vi "Fetch_Source.vi"(8 "error in (no error)":errorcluster, 9 "destTag":string, 10 "sourceTag":string, 11 "Installer in":refnum<class "Installer.lvclass">) -> (0 "error out":errorcluster, 2 "index":i32, 3 "IB_Source.lvclass":refnum<class "IB_Source.lvclass">)   [LabVIEW 2020, in "Installer.lvclass"]
uses:
  <vilib>/AppBuilder/IB_Classes/Installer/Installer.lvclass
  <vilib>/AppBuilder/IB_Classes/Installer/Installer.lvclass/Installer.ctl
  <vilib>/AppBuilder/IB_Classes/Source/IB_Source.lvclass
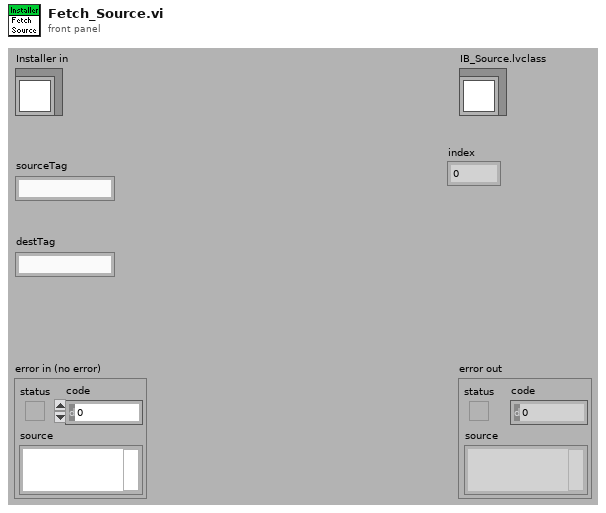
[diagram p1: front panel]
types:
  T1 = typedef "IB_Source.ctl" = cluster{"name":string, "sourceTag":string, "destTag":string, "path":path, "eng_installPath":string, "UI_inBuild?":bool, "str ref?":bool}
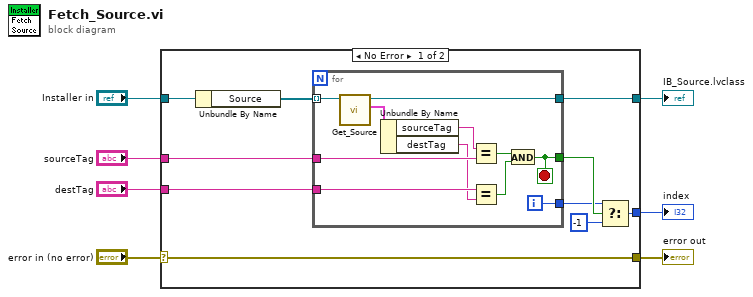
[diagram p0: block diagram]
diagram:
  n1 = case shown="No Error" "error in (no error)" {
    selector: "error in (no error)" -> [w17 w29]
    tunnel: [w17 w29] -> w6
    tunnel: "Installer in" -> [w16 _]
    tunnel: [w14 _] -> w4
    tunnel: "sourceTag" -> [w13 _]
    tunnel: "destTag" -> [w12 _]
    tunnel: [w8 _] -> w1
    frame No Error {
      n2 = Unbundle By Name(w16) -> ("Source"=w15:refnum<class "IB_Source.lvclass">[])
      n3 = for {
        tunnel: w15 -> [w28] mode=indexing
        tunnel: [w27] -> w14
        tunnel: w13 -> [w24]
        tunnel: w12 -> [w23]
        tunnel: [w19] -> w11
        tunnel: [w18] -> w10
        i -> [w18]
        stop <- w19 stop-if-true
        n4 = call <vilib>:"Get_Source.vi"("IB_Source in"=w28) -> ("data"=w26:T1, "IB_Source out"=w27:refnum<class "IB_Source.lvclass">)  [unwired: 8 in, 1 out]
        n5 = Unbundle By Name(w26) -> ("sourceTag"=w25:string, "destTag"=w22:string)
        n6 = Equal?(x=w25, y=w24) -> (x = y?=w21:bool)
        n7 = Equal?(x=w23, y=w22) -> (x = y?=w20:bool)
        n8 = And(x=w21, y=w20) -> (x .and. y?=w19:bool)
      }
      n9 = Select(t=w10, s=w11, f=-1) -> (s? t:f=w8:i32)
    }
    frame Error {
    }
  }
  "error out" <- w6
  "IB_Source.lvclass" <- w4
  "index" <- w1
